vi "laserzzzz.vi"(2 "Yin":i32, 3 "Xin":i32) -> (0 "Angle Y":dbl, 1 "Angle X":dbl)   [LabVIEW 2014]
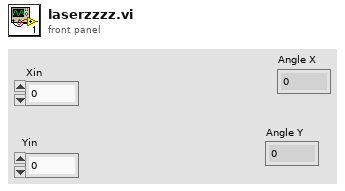
[diagram p1: front panel]
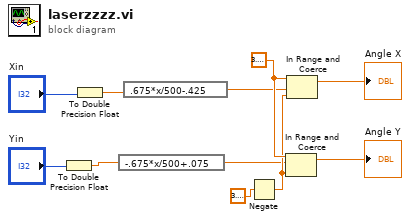
[diagram p0: block diagram]
diagram:
  w8 = 3.141592653589793
  n1 = To Double Precision Float(number="Yin") -> (double precision float=w7:dbl)
  n2 = To Double Precision Float(number="Xin") -> (double precision float=w9:dbl)
  n3 = expression code="-.675*x/500+.075"(w7) -> (w1:dbl)
  n4 = expression code=".675*x/500-.425"(w9) -> (w2:dbl)
  n5 = Negate(x=3.141592653589793) -> (-x=w3:dbl)
  n6 = In Range and Coerce(upper limit=w8, x=w1, lower limit=w3) -> (coerced(x)=→"Angle Y":dbl)  [unwired: 1 out]
  n7 = In Range and Coerce(upper limit=w8, x=w2, lower limit=w3) -> (coerced(x)=→"Angle X":dbl)  [unwired: 1 out]
